vi "Measurement Logic.vi"() -> ()   [LabVIEW 2020, in "NIScopeAcquireWaveform.lvlib"]
uses:
  NIScopeAcquireWaveform.lvlib
  Measurement Results.ctl
  <vilib>/MeasurementLink/MeasurementLink Measurement Server/Measure Call Context/Measure Call Context.lvclass
  <vilib>/MeasurementLink/MeasurementLink niScope/Initialize Sessions - 1Sess.vi
  <vilib>/MeasurementLink/MeasurementLink niScope/Get Connections - NPin MConn.vi
  <vilib>/MeasurementLink/MeasurementLink niScope/Get Connections - 1Pin 1Conn.vi
  <instrlib>/niScope/Configure/Trigger/niScope Configure Trigger Edge.vi
  <instrlib>/niScope/Acquire/Fetch/niScope Multi Fetch WDT.vi
  <vilib>/MeasurementLink/MeasurementLink niScope/MeasurementLink niScope.lvlib
  <vilib>/MeasurementLink/MeasurementLink Session Management V1/Session Reservation/Session Reservation.lvclass
  <instrlib>/niScope/Controls/niScope vertical coupling.ctl
  <instrlib>/niScope/Controls/niScope trigger slope.ctl
  Measurement Configuration.ctl
panel:
  in  "measurement configuration":T1={"Pin Names"=["PinGroup1"], "Vertical Range"=5.0, "Vertical Coupling"=1, "Input Impedance"=0, "Minimum Sample Rate"=10000000.0, "Minimum Record Length"=40000, "Trigger Source"="Pin1", "Trigger Level"=0.5, "Trigger Slope"=0, "Timeout"=5.0, "Trigger Coupling"=1} {"Input Impedance" items=["1 mega ohm"=0, "50 ohms"=2]; "Trigger Coupling" items=["AC"=0, "DC"=1, "HF Reject"=3, "LF Reject"=4, "AC Plus HF Reject"=1001]; "Trigger Slope" items=["Positive", "Negative"]; "Vertical Coupling" items=["AC", "DC", "Ground"]}
  out "measure call context out":refnum<class "Measure Call Context.lvclass">
  in  "measure call context in":refnum<class "Measure Call Context.lvclass">
  out "measurement results":T4
  out "error out":errorcluster
  in  "error in":errorcluster
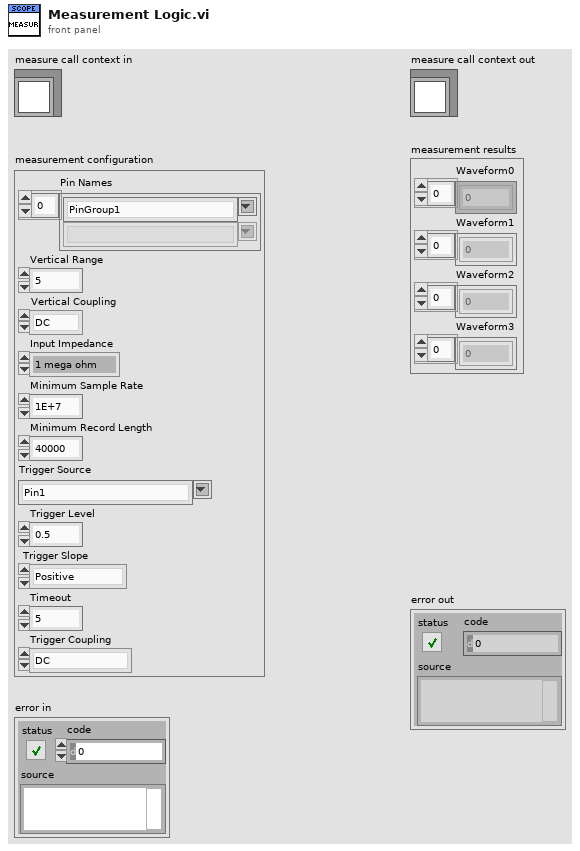
[diagram p1: front panel]
types:
  T1 = typedef "NIScopeAcquireWaveform.lvlib/Measurement Configuration.ctl" = cluster{"Pin Names":string[], "Vertical Range":dbl, "Vertical Coupling":T2, "Input Impedance":u32, "Minimum Sample Rate":dbl, "Minimum Record Length":i32, "Trigger Source":string, "Trigger Level":dbl, "Trigger Slope":T3, "Timeout":dbl, "Trigger Coupling":u32}
  T2 = typedef "niScope vertical coupling.ctl" = i32
  T3 = typedef "niScope trigger slope.ctl" = i32
  T4 = typedef "NIScopeAcquireWaveform.lvlib/Measurement Results.ctl" = cluster{"Waveform0":dbl[], "Waveform1":dbl[], "Waveform2":dbl[], "Waveform3":dbl[]}
  T5 = typedef "MeasurementLink niScope.lvlib/Connection with Session.ctl" = cluster{"connection":T6, "session":refnum<k15>}
  T6 = typedef "MeasurementLink Session Management V1.lvlib/Session Reservation.lvclass/Connection.ctl" = cluster{"pin or relay name":string, "site":i32, "instrument type id":string, "channel":string}
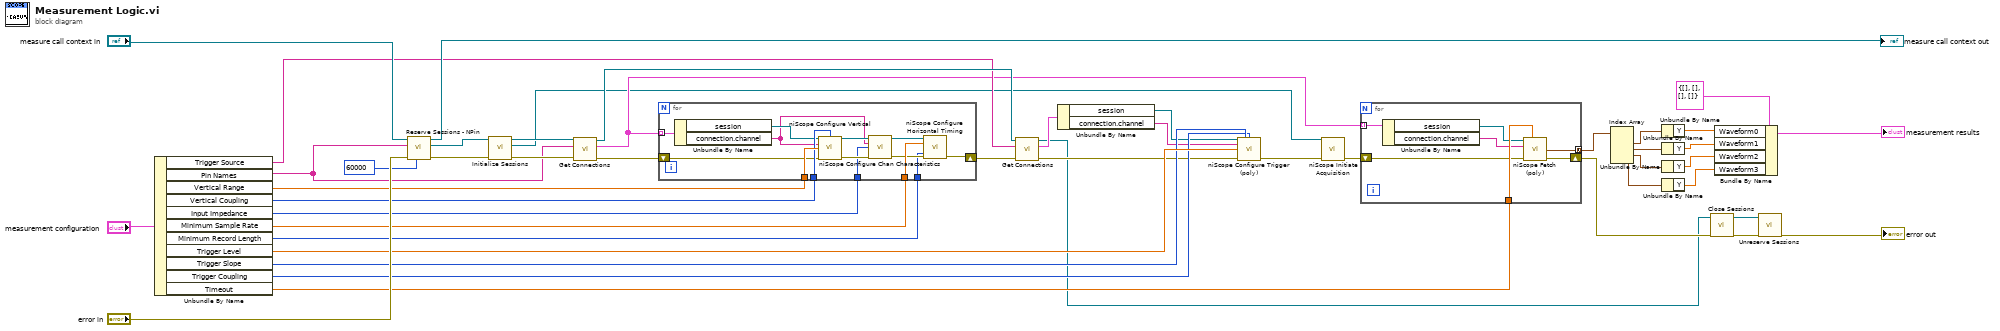
[diagram p0: block diagram]
diagram:
  n1 = Unbundle By Name("measurement configuration") -> ("Trigger Source"=w8:string, "Pin Names"=w2:string[], "Vertical Range"=w40:dbl, "Vertical Coupling"=w29:T2, "Input Impedance"=w21:u32, "Minimum Sample Rate"=w17:dbl, "Minimum Record Length"=w16:i32, "Trigger Level"=w39:dbl, "Trigger Slope"=w28:T3, "Trigger Coupling"=w27:u32, "Timeout"=w26:dbl)
  n2 = call <vilib>:"Reserve Sessions - NPin.vi"("timeout (ms)"=60000, "error in"="error in", "pin or relay names"=w2, "measurement context in"="measure call context in") -> ("error out"=w41:errorcluster, "session reservation out"=w42:refnum<class "Session Reservation.lvclass">, "measurement context out"=→"measure call context out":refnum<class "Measure Call Context.lvclass">)  [unwired: 5 in]
  n3 = call-poly <vilib>:"Initialize Sessions.vi"("error in"=w41, "session reservation in"=w42) -> ("error out"=w20:errorcluster, "session"=w4:refnum<k15>, "session reservation out"=w19:refnum<class "Session Reservation.lvclass">)  [unwired: 6 in, 1 out]
  n4 = call-poly <vilib>:"Get Connections.vi"("error in"=w20, "pin or relay names"=w2, "session reservation in"=w19) -> ("error out"=w18:errorcluster, "connections"=w7:T5[], "session reservation out"=w13:refnum<class "Session Reservation.lvclass">)  [unwired: 6 in]
  n5 = for {
    tunnel: w40 -> [w60]
    tunnel: w29 -> [w58]
    tunnel: w21 -> [w57]
    shift-right: [w49] -> w15
    shift-left: w18 -> [w56]
    tunnel: w7 -> [w55] mode=indexing
    tunnel: w17 -> [w53]
    tunnel: w16 -> [w51]
    n6 = Unbundle By Name(w55) -> ("session"=w54:refnum<k15>, "connection.channel"=w48:string)
    n7 = call <instrlib>:"niScope Configure Vertical.vi"("instrument handle"=w54, "vertical coupling"=w58, "channels"=w48, "vertical range"=w60, "error in"=w56) -> ("instrument handle out"=w61:refnum<k15>, "error out"=w59:errorcluster)  [unwired: 9 in]
    n8 = call <instrlib>:"niScope Configure Chan Characteristics.vi"("instrument handle"=w61, "channels"=w48, "input impedance"=w57, "error in"=w59) -> ("instrument handle out"=w50:refnum<k15>, "error out"=w52:errorcluster)  [unwired: 10 in]
    n9 = call <instrlib>:"niScope Configure Horizontal Timing.vi"("instrument handle"=w50, "min sample rate"=w53, "error in"=w52, "min record length"=w51) -> ("error out"=w49:errorcluster)  [unwired: 10 in, 1 out]
  }
  n10 = call-poly <vilib>:"Get Connections.vi"("error in"=w15, "pin or relay name"=w8, "session reservation in"=w13) -> ("error out"=w14:errorcluster, "connection"=w12:T5, "session reservation out"=w9:refnum<class "Session Reservation.lvclass">)  [unwired: 6 in]
  n11 = Unbundle By Name(w12) -> ("session"=w11:refnum<k15>, "connection.channel"=w10:string)
  n12 = call-poly <instrlib>:"niScope Configure Trigger (poly).vi"("instrument handle"=w11, "trigger slope"=w28, "trigger coupling"=w27, "trigger source"=w10, "trigger level"=w39, "error in"=w14) -> ("error out"=w5:errorcluster)  [unwired: 8 in, 1 out]
  n13 = call <instrlib>:"niScope Initiate Acquisition.vi"("instrument handle"=w4, "error in"=w5) -> ("error out"=w6:errorcluster)  [unwired: 12 in, 1 out]
  n14 = for {
    tunnel: [w68] -> w38 mode=concatenating
    tunnel: w26 -> [w67]
    shift-right: [w66] -> w23
    shift-left: w6 -> [w62]
    tunnel: w7 -> [w65] mode=indexing
    n15 = Unbundle By Name(w65) -> ("session"=w64:refnum<k15>, "connection.channel"=w63:string)
    n16 = call-poly <instrlib>:"niScope Fetch (poly).vi"("timeout"=w67, "error in"=w62, "channels"=w63, "instrument handle"=w64) -> ("error out"=w66:errorcluster, "wfm"=w68:waveform(dbl)[])  [unwired: 4 in, 2 out]
  }
  n17 = Index Array(array=w38) -> (element #1=w33:waveform(dbl), element #2=w32:waveform(dbl), element #3=w31:waveform(dbl), element #4=w30:waveform(dbl))  [unwired: 4 in]
  n18 = Unbundle By Name(w33) -> ("Y"=w37:dbl[])
  n19 = Unbundle By Name(w32) -> ("Y"=w36:dbl[])
  n20 = Unbundle By Name(w31) -> ("Y"=w35:dbl[])
  n21 = Unbundle By Name(w30) -> ("Y"=w34:dbl[])
  n22 = call <vilib>:"Close Sessions.vi"("error in"=w23, "session reservation in"=w9) -> ("error out"=w24:errorcluster, "session reservation out"=w22:refnum<class "Session Reservation.lvclass">)  [unwired: 8 in]
  n23 = Bundle By Name(cluster=T4 {"Waveform0"=[], "Waveform1"=[], "Waveform2"=[], "Waveform3"=[]} ("Measurement Results"), "Waveform0"=w37, "Waveform1"=w36, "Waveform2"=w35, "Waveform3"=w34) -> (→"measurement results":T4)
  n24 = call <vilib>:"Unreserve Sessions.vi"("error in"=w24, "session reservation in"=w22) -> ("error out"=→"error out":errorcluster)  [unwired: 9 in]
